vi "Client UI.vi"() -> ()   [LabVIEW 2020, in "LV Chat Client.lvclass"]
uses:
  LV Chat Client.lvclass
  UI State.ctl
  Data Types/Message.ctl
  LV Chat Client.lvclass/LV Chat Client.ctl
  <vilib>/IlluminatedG/lv-msg-simple/Stream-Simple-Msg/Manager/Manager.lvclass
  Data Types/Message ID.ctl
  <vilib>/event_ctls.llb/eventvkey.ctl
  Events.ctl
  <vilib>/IlluminatedG/lv-stream/Connection State.ctl
  Data Types/User Info.ctl
  01a2a97e-4748-4b48-9309-911c4d3a1048.vi
  b7fc8858-76c6-4de5-805f-2f843daa277e.vi
  b7fc8858-76c6-4de5-805f-2f843daa277e.vi/43e93f4b-eb60-4448-b7e4-56a49cc750fb.vi
  b7fc8858-76c6-4de5-805f-2f843daa277e.vi/0bdc4188-3073-475f-bdb7-d424a9377977.vi
  <vilib>/IlluminatedG/lv-msg-simple/Stream-Simple-Msg/Message/_Create.vi
  <vilib>/IlluminatedG/lv-msg-simple/Stream-Simple-Msg/Manager/Get Endpoints.vi
  <vilib>/IlluminatedG/lv-msg-simple/Stream-Simple-Msg/Message/Get Flattened Message.vi
  <vilib>/IlluminatedG/lv-msg-simple/Stream-Simple-Msg/Endpoint/Get Stream.vi
  <vilib>/IlluminatedG/lv-msg-simple/Stream-Simple-Msg/Message/Message.lvclass
  <vilib>/IlluminatedG/lv-stream/stream/Stream.lvclass
  <vilib>/IlluminatedG/lv-stream/Stream.lvlib
panel:
  in  "Timestamps":bool
  out "# Users":i32
  in  "Disconnect":bool
  in  "Connect":bool
  out "Log":string
  out "Users":i32(listbox)
  in  "Send":bool
  in  "Text":string
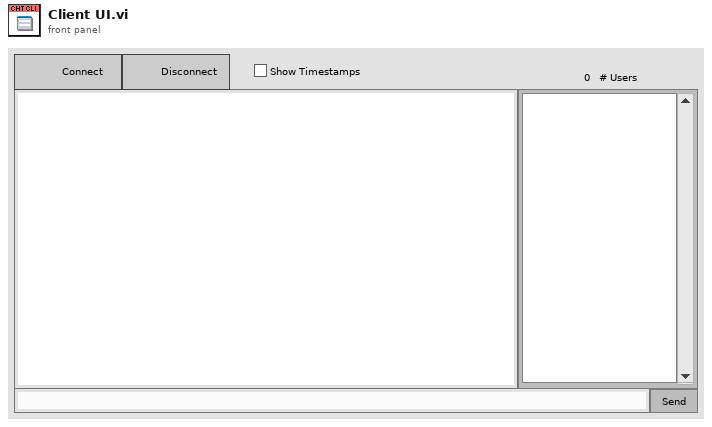
[diagram p1: front panel]
types:
  T1 = typedef "LV Chat Client.lvclass/UI State.ctl" = enum16{"Init", "Run", "Close"}
  T2 = typedef "Message.ctl" = cluster{"From":string, "Time":dbl, "Message":string}
  T3 = enum8{"Enabled", "Disabled", "Disabled and Grayed Out"}
  T4 = typedef "Message ID.ctl" = enum16{"UserInfo", "UserList", "Message", "Disconnect"}
  T5 = typedef "eventvkey.ctl" = enum16{"ASCII", "Enter", "Return", "Shift", "Ctrl", "Alt", "Cmd", "Opt", "Caps", "NumLock", "Clear", "Break", "Up", "Down", "Left", "Right", "Insert", "Delete", "Home", "End", "PageUp", "PageDown", "Escape", "Help", "Pause", "ScrollLock", "F1", "F2", "F3", "F4", "F5", "F6", "F7", "F8", "F9", "F10", "F11", "F12", "F13", "F14", "F15", "F16", "F17", "F18", "F19", "F20", "F21", "F22", "F23", "F24", "Play", "VolumeUp", "VolumeDown", "Mute", "Two Byte Char"}
  T6 = typedef "LV Chat Client.lvclass/Events.ctl" = cluster{"Userlist":refnum<user-event>, "Message":refnum<user-event>, "Prompt Name":refnum<user-event>, "Connection":refnum<user-event>, "Userinfo":refnum<user-event>, "Log":refnum<user-event>, "Update Log":refnum<user-event>}
  T7 = typedef "Stream.lvlib/Connection State.ctl" = enum16{"Connected", "Disconnected"}
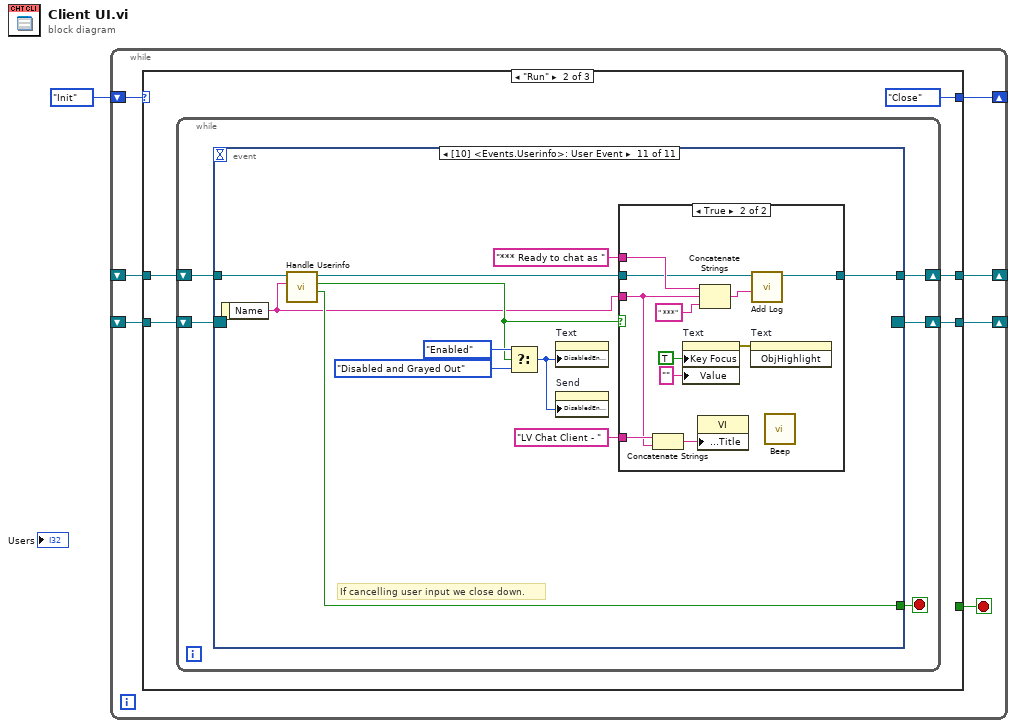
[diagram p0: block diagram]
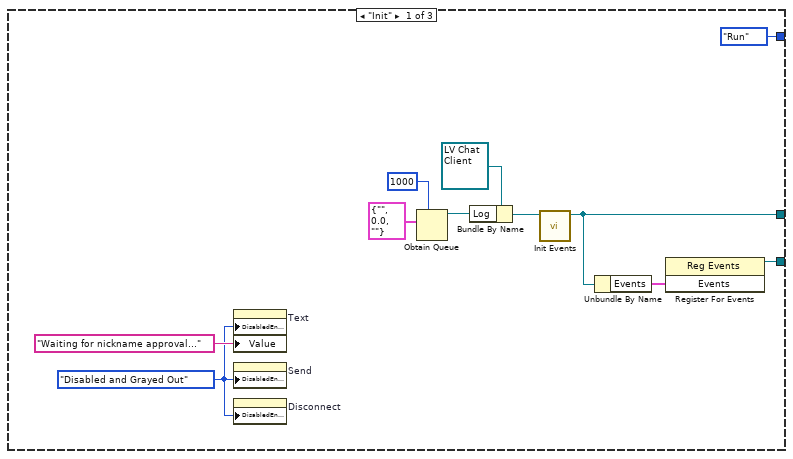
[diagram p2: hidden frame]
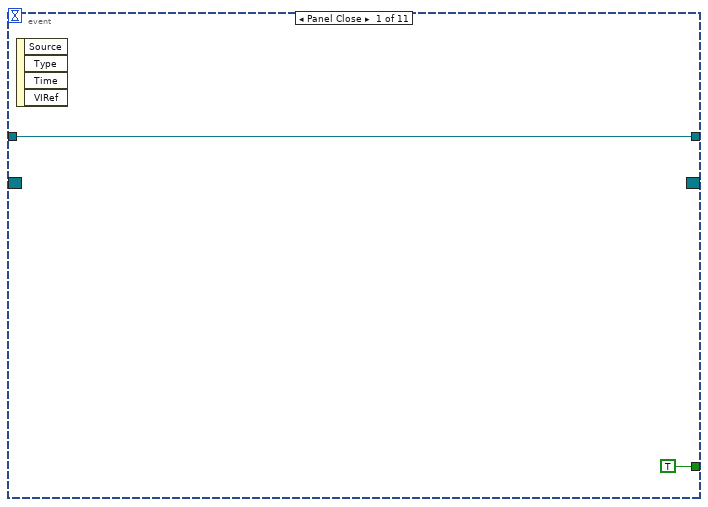
[diagram p3: hidden frame]
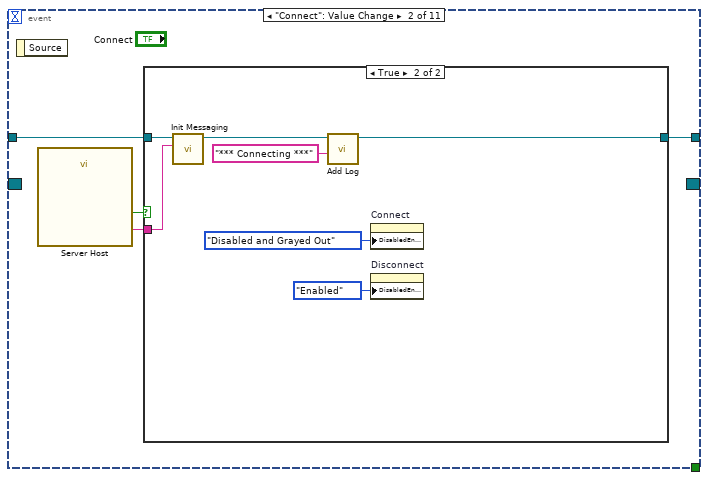
[diagram p4: hidden frame]
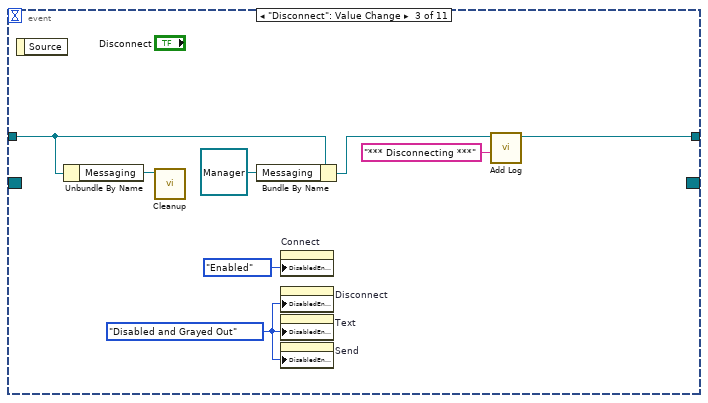
[diagram p6: hidden frame]
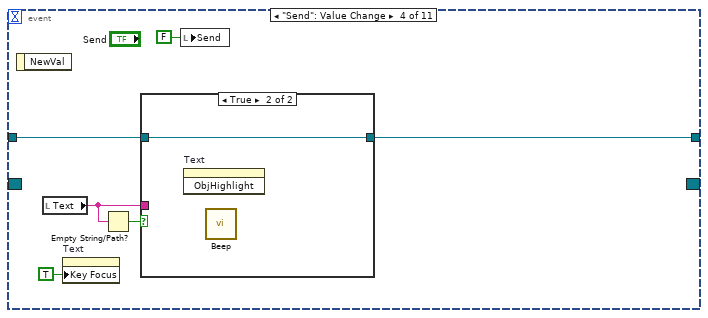
[diagram p7: hidden frame]
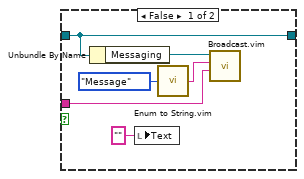
[diagram p8: hidden frame]
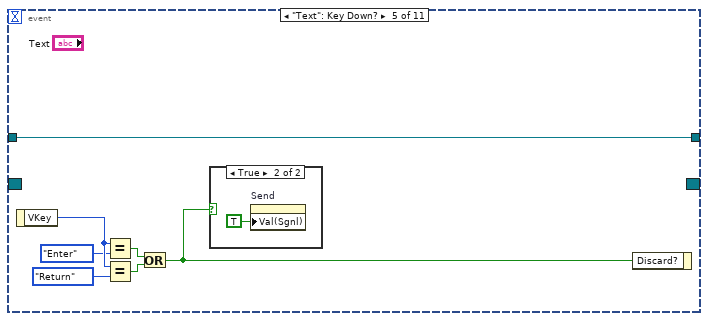
[diagram p9: hidden frame]
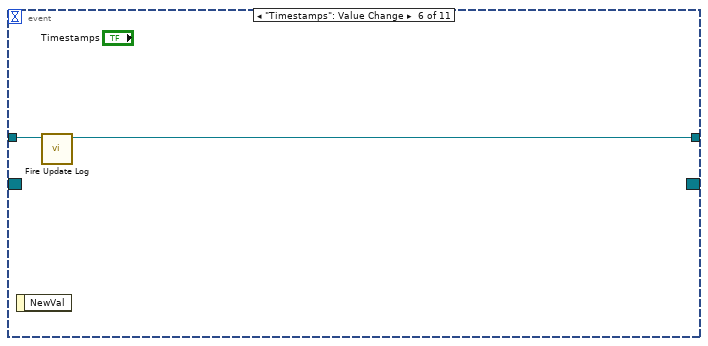
[diagram p11: hidden frame]
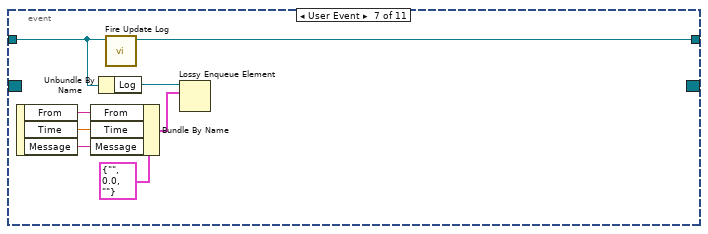
[diagram p12: hidden frame]
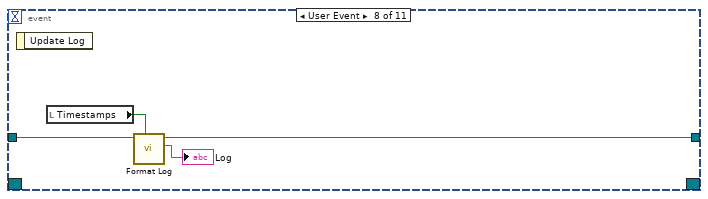
[diagram p13: hidden frame]
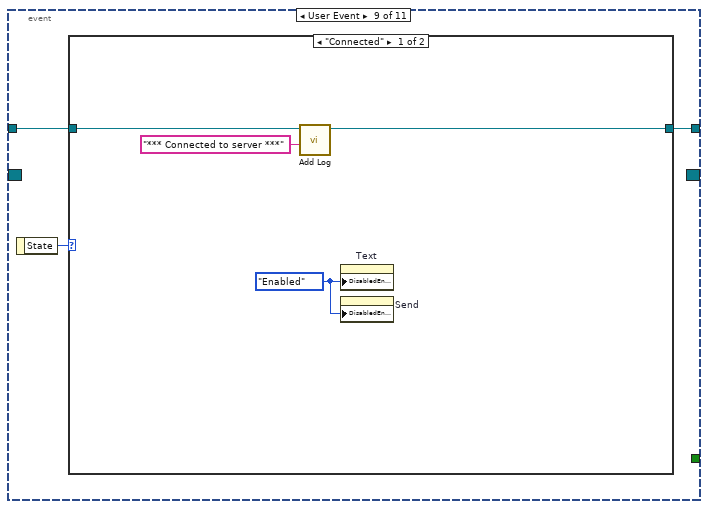
[diagram p14: hidden frame]
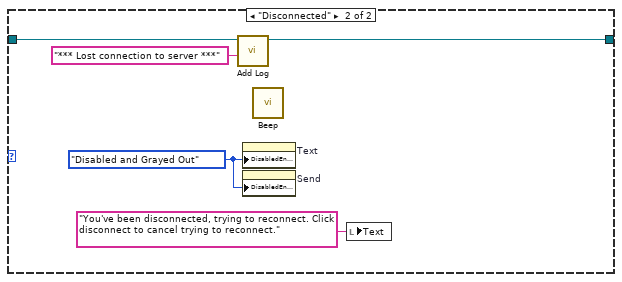
[diagram p15: hidden frame]
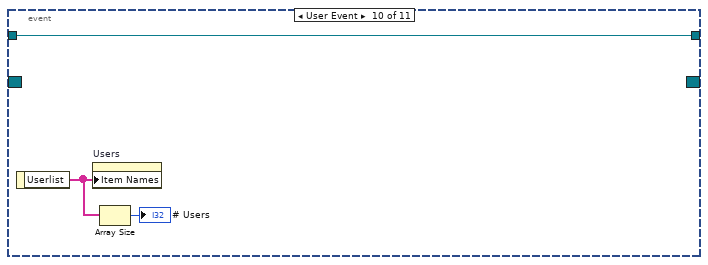
[diagram p16: hidden frame]
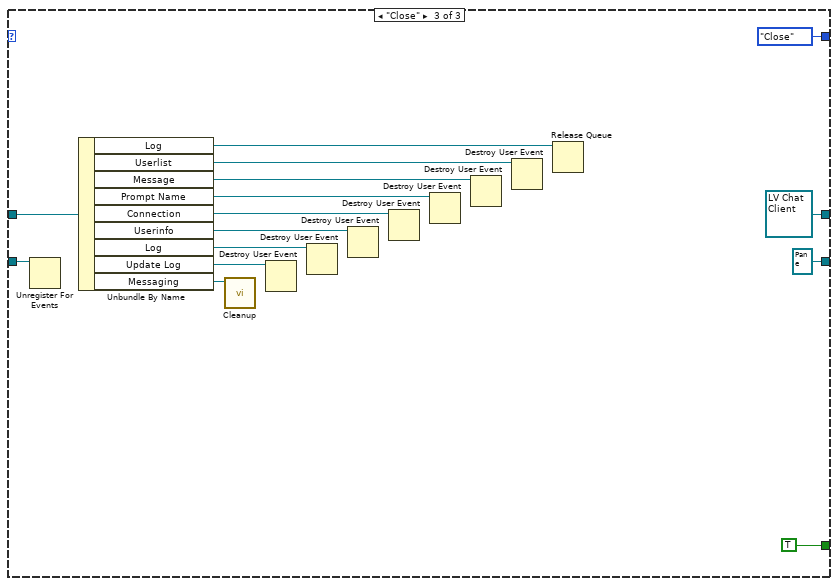
[diagram p18: hidden frame]
diagram:
  n1 = while {
    shift-right: [w5] -> _
    shift-left: UI_State."Init" ("UI State") -> [w8]
    shift-right: [w4] -> _
    shift-left: _ -> [w7]
    shift-right: [w3] -> _
    shift-left: _ -> [w2]
    stop <- w6 stop-if-true
    n2 = case shown="\"Run\"" w8 {
      tunnel: w7 -> [_ w23 w134]
      tunnel: [_ _ TRUE] -> w6
      tunnel: [UI_State."Run" ("UI State") UI_State."Close" ("UI State") UI_State."Close" ("UI State")] -> w5
      tunnel: [w13 w22 refnum<class "LV Chat Client.lvclass"> refnum ("LV Chat Client out")] -> w4
      tunnel: [w17 w20 refnum<event-registration> refnum ("Event Registration Refnum")] -> w3
      tunnel: w2 -> [_ w21 w136]
      frame "Init" {
        w15 = T3."Disabled and Grayed Out" ("Disabled")
        n3 = property on="Text" class="Str"("DisabledEnum"=w15, "Value"="Waiting for nickname approval..." ("Text")) -> ()  [unwired: 2 in, 2 out]
        n4 = property on="Send" class="Bool (strict)"("DisabledEnum"=w15) -> ()  [unwired: 2 in, 2 out]
        n5 = property on="Disconnect" class="Bool"("DisabledEnum"=w15) -> ()  [unwired: 2 in, 2 out]
        n6 = Obtain Queue(max queue size (-1, unlimited)=1000, element data type=T2 {"From"="", "Time"=0.0, "Message"=""} ("Message")) -> (queue out=w9:refnum<queue>)  [unwired: 3 in, 2 out]
        n7 = Bundle By Name(cluster=refnum<class "LV Chat Client.lvclass"> refnum ("LV Chat Client out"), "Log"=w9) -> (w12:refnum<class "LV Chat Client.lvclass">)
        n8 = call "Init Events.vi"("LV Chat Client in"=w12) -> ("LV Chat Client out"=w13:refnum<class "LV Chat Client.lvclass">)  [unwired: 9 in, 1 out]
        n9 = Unbundle By Name(w13) -> ("Events"=w18:T6)
        n10 = register-events(w18) -> (reference out=w17:refnum<event-registration>)  [unwired: 2 in, 1 out]
      }
      frame "Run" {
        n11 = while {
          shift-right: [w27] -> w22
          shift-left: w23 -> [w28]
          shift-right: [w25] -> w20
          shift-left: w21 -> [w26]
          stop <- w29 stop-if-true
          n12 = event shown="[10] <Events.Userinfo>: User Event" {
            selector: w26 -> [_ _ _ _ _ _ _ _ _ _ _]
            dyn-events: [_ _ _ _ _ _ _ _ _ _ _] -> w25
            timeout: _ -> [_ _ _ _ _ _ _ _ _ _ _]
            tunnel: [TRUE _ _ _ _ _ _ _ _ _ w111] -> w29
            tunnel: w28 -> [w30 w34 w49 w54 w65 w74 w76 w86 w88 w99 w112]
            tunnel: [w30 w32 w45 w53 w65 w73 w75 w84 w87 w99 w104] -> w27
            event Panel Close {
              n13 = event-data() -> ()  [unwired: 1 in, 4 out]
            }
            event "Connect": Value Change {
              n14 = event-data() -> ()  [unwired: 1 in, 1 out]
              n15 = call "Server Host"() -> ("Server Host"=w33:string, "OK"=w35:bool)  [unwired: 17 in, 1 out]
              n16 = case shown="True" w35 {
                tunnel: w34 -> [w36 w43]
                tunnel: w33 -> [_ w42]
                tunnel: [w36 w37] -> w32
                frame False {
                }
                frame True {
                  n17 = call "Init Messaging.vi"("Server Host"=w42, "LV Chat Client in"=w43) -> ("LV Chat Client out"=w39:refnum<class "LV Chat Client.lvclass">)  [unwired: 8 in, 1 out]
                  n18 = call "Add Log.vi"("Message"="*** Connecting ***", "LV Chat Client in"=w39) -> ("LV Chat Client out"=w37:refnum<class "LV Chat Client.lvclass">)  [unwired: 8 in, 1 out]
                  n19 = property on="Connect" class="Bool"("DisabledEnum"=T3."Disabled and Grayed Out" ("Disabled")) -> ()  [unwired: 2 in, 2 out]
                  n20 = property on="Disconnect" class="Bool"("DisabledEnum"=T3."Enabled" ("Disabled")) -> ()  [unwired: 2 in, 2 out]
                }
              }
            }
            event "Disconnect": Value Change {
              w47 = T3."Disabled and Grayed Out" ("Disabled")
              n21 = event-data() -> ()  [unwired: 1 in, 1 out]
              n22 = Unbundle By Name(w49) -> ("Messaging"=w50:refnum<class "Manager.lvclass">)
              n23 = call <vilib>:"Cleanup.vi"("Manager in"=w50) -> ()  [unwired: 10 in, 1 out]
              n24 = Bundle By Name(cluster=w49, "Messaging"=refnum<class "Manager.lvclass"> refnum) -> (w46:refnum<class "LV Chat Client.lvclass">)
              n25 = property on="Connect" class="Bool"("DisabledEnum"=T3."Enabled" ("Disabled")) -> ()  [unwired: 2 in, 2 out]
              n26 = property on="Disconnect" class="Bool"("DisabledEnum"=w47) -> ()  [unwired: 2 in, 2 out]
              n27 = property on="Text" class="Str"("DisabledEnum"=w47) -> ()  [unwired: 2 in, 2 out]
              n28 = property on="Send" class="Bool (strict)"("DisabledEnum"=w47) -> ()  [unwired: 2 in, 2 out]
              n29 = call "Add Log.vi"("Message"="*** Disconnecting ***", "LV Chat Client in"=w46) -> ("LV Chat Client out"=w45:refnum<class "LV Chat Client.lvclass">)  [unwired: 8 in, 1 out]
            }
            event "Send": Value Change {
              n30 = event-data() -> ()  [unwired: 1 in, 1 out]
              n31 = local read "Text"() -> (w55:string)
              n32 = property on="Text" class="Str"("Key Focus"=TRUE) -> ()  [unwired: 2 in, 2 out]
              n33 = Empty String/Path?(string/path=w55) -> (empty?=w56:bool)
              n34 = case shown="True" w56 {
                tunnel: w55 -> [w60 _]
                tunnel: w54 -> [w62 w64]
                tunnel: [w62 w64] -> w53
                frame False {
                  n35 = Unbundle By Name(w62) -> ("Messaging"=w61:refnum<class "Manager.lvclass">)
                  n36 = local write "Text"("" ("Text")) -> ()
                  n37 = call "Enum to String.vim"("Enum"=Message_ID."Message" ("Message ID")) -> ("Enum String"=w58:string)
                  n38 = call "Broadcast.vim"("Data (With ID String)"=w60, "Message (Or ID String)"=w58, "Manager in"=w61) -> ()  [unwired: 7 in, 2 out]
                }
                frame True {
                  n39 = invoke on="Text" class="Str" method="ObjHighlight"() -> ()  [unwired: 3 in, 3 out]
                  n40 = call <vilib>:"Beep.vi"() -> ()  [unwired: 12 in]
                }
              }
              n41 = local write "Send"(FALSE ("Send")) -> ()
            }
            event "Text": Key Down? {
              n42 = event-data() -> ("VKey"=w71:T5)  [unwired: 1 in]
              n43 = Equal?(x=w71, y=eventvkey."Enter") -> (x = y?=w68:bool)
              n44 = Equal?(x=w71, y=eventvkey."Return") -> (x = y?=w67:bool)
              n45 = Or(x=w68, y=w67) -> (x .or. y?=w66:bool)
              n46 = case shown="True" w66 {
                frame False {
                }
                frame True {
                  n47 = property on="Send" class="Bool (strict)"("Val(Sgnl)"=TRUE ("Value (Signaling)")) -> ()  [unwired: 2 in, 2 out]
                }
              }
              n48 = event-data("Discard?"=w66) -> ()  [unwired: 1 in, 1 out]
            }
            event "Timestamps": Value Change {
              n49 = event-data() -> ()  [unwired: 1 in, 1 out]
              n50 = call "Fire Update Log.vi"("LV Chat Client in"=w74) -> ("LV Chat Client out"=w73:refnum<class "LV Chat Client.lvclass">)  [unwired: 9 in, 1 out]
            }
            event User Event {
              n51 = event-data() -> ("From"=w81:string, "Time"=w80:dbl, "Message"=w79:string)  [unwired: 1 in]
              n52 = Bundle By Name(cluster=T2 {"From"="", "Time"=0.0, "Message"=""} ("Message"), "From"=w81, "Time"=w80, "Message"=w79) -> (w77:T2)
              n53 = Unbundle By Name(w76) -> ("Log"=w78:refnum<queue>)
              n54 = call "Fire Update Log.vi"("LV Chat Client in"=w76) -> ("LV Chat Client out"=w75:refnum<class "LV Chat Client.lvclass">)  [unwired: 9 in, 1 out]
              n55 = Lossy Enqueue Element(queue=w78, element=w77) -> ()  [unwired: 1 in, 4 out]
            }
            event User Event {
              n56 = event-data() -> ()  [unwired: 1 in, 1 out]
              n57 = local read "Timestamps"() -> (w85:bool)
              n58 = call "Format Log.vi"("Show Timestamps"=w85, "LV Chat Client in"=w86) -> ("Log"=→"Log":string, "LV Chat Client out"=w84:refnum<class "LV Chat Client.lvclass">)  [unwired: 7 in, 1 out]
            }
            event User Event {
              n59 = event-data() -> ("State"=w89:T7)  [unwired: 1 in]
              n60 = case shown="\"Connected\"" w89 {
                tunnel: w88 -> [w92 w96]
                tunnel: [w90 w94] -> w87
                frame "Connected" {
                  w93 = T3."Enabled" ("Disabled")
                  n61 = call "Add Log.vi"("Message"="*** Connected to server ***", "LV Chat Client in"=w92) -> ("LV Chat Client out"=w90:refnum<class "LV Chat Client.lvclass">)  [unwired: 8 in, 1 out]
                  n62 = property on="Text" class="Str"("DisabledEnum"=w93) -> ()  [unwired: 2 in, 2 out]
                  n63 = property on="Send" class="Bool (strict)"("DisabledEnum"=w93) -> ()  [unwired: 2 in, 2 out]
                }
                frame "Disconnected" {
                  w98 = T3."Disabled and Grayed Out" ("Disabled")
                  n64 = call "Add Log.vi"("Message"="*** Lost connection to server ***", "LV Chat Client in"=w96) -> ("LV Chat Client out"=w94:refnum<class "LV Chat Client.lvclass">)  [unwired: 8 in, 1 out]
                  n65 = property on="Text" class="Str"("DisabledEnum"=w98) -> ()  [unwired: 2 in, 2 out]
                  n66 = property on="Send" class="Bool (strict)"("DisabledEnum"=w98) -> ()  [unwired: 2 in, 2 out]
                  n67 = call <vilib>:"Beep.vi"() -> ()  [unwired: 12 in]
                  n68 = local write "Text"("You've been disconnected, trying to reconnect. Click disconnect to cancel trying to reconnect." ("Text")) -> ()
                }
              }
            }
            event User Event {
              n69 = event-data() -> ("Userlist"=w101:string[])  [unwired: 1 in]
              n70 = property on="Users" class="LstBox (strict)"("Item Names"=w101) -> ()  [unwired: 2 in, 2 out]
              n71 = Array Size(array=w101) -> (size(s)=→"# Users":i32)
            }
            event User Event {
              # "If cancelling user input we close down."
              n72 = event-data() -> ("Name"=w106:string)  [unwired: 1 in]
              n73 = call "Handle Userinfo.vi"("Name"=w106, "LV Chat Client in"=w112) -> ("Cancelled?"=w111:bool, "Name Accepted?"=w108:bool, "LV Chat Client out"=w107:refnum<class "LV Chat Client.lvclass">)  [unwired: 6 in, 1 out]
              n74 = Select(t=T3."Enabled" ("Disabled"), s=w108, f=T3."Disabled and Grayed Out" ("Disabled")) -> (s? t:f=w103:T3)
              n75 = property on="Text" class="Str"("DisabledEnum"=w103) -> ()  [unwired: 2 in, 2 out]
              n76 = property on="Send" class="Bool (strict)"("DisabledEnum"=w103) -> ()  [unwired: 2 in, 2 out]
              n77 = case shown="True" w108 {
                tunnel: w107 -> [w113 w119]
                tunnel: w106 -> [_ w115]
                tunnel: "*** Ready to chat as " -> [_ w121]
                tunnel: [w113 w117] -> w104
                tunnel: "LV Chat Client - " -> [_ w116]
                frame False {
                }
                frame True {
                  n78 = Concatenate Strings(w116, w115) -> (w114:string)
                  n79 = property on="Text" class="Str"("Key Focus"=TRUE, "Value"="" ("Text")) -> (error out=w123:errorcluster)  [unwired: 2 in, 1 out]
                  n80 = property class="VI"("Front Panel.Title"=w114) -> ()  [unwired: 2 in, 2 out]
                  n81 = Concatenate Strings(w121, w115, " ***" ("string")) -> (w118:string)
                  n82 = invoke on="Text" class="Str" method="ObjHighlight"(error in=w123) -> ()  [unwired: 2 in, 3 out]
                  n83 = call "Add Log.vi"("Message"=w118, "LV Chat Client in"=w119) -> ("LV Chat Client out"=w117:refnum<class "LV Chat Client.lvclass">)  [unwired: 8 in, 1 out]
                  n84 = call <vilib>:"Beep.vi"() -> ()  [unwired: 12 in]
                }
              }
            }
          }
        }
      }
      frame "Close" {
        n85 = Unregister For Events(event registration refnum=w136) -> ()  [unwired: 1 in, 1 out]
        n86 = Unbundle By Name(w134) -> ("Log"=w125:refnum<queue>, "Userlist"=w126:refnum<user-event>, "Message"=w127:refnum<user-event>, "Prompt Name"=w128:refnum<user-event>, "Connection"=w129:refnum<user-event>, "Userinfo"=w130:refnum<user-event>, "Log"=w131:refnum<user-event>, "Update Log"=w132:refnum<user-event>, "Messaging"=w133:refnum<class "Manager.lvclass">)
        n87 = call <vilib>:"Cleanup.vi"("Manager in"=w133) -> ()  [unwired: 10 in, 1 out]
        n88 = Destroy User Event(user event=w132) -> ()  [unwired: 1 in, 1 out]
        n89 = Destroy User Event(user event=w131) -> ()  [unwired: 1 in, 1 out]
        n90 = Destroy User Event(user event=w130) -> ()  [unwired: 1 in, 1 out]
        n91 = Destroy User Event(user event=w129) -> ()  [unwired: 1 in, 1 out]
        n92 = Destroy User Event(user event=w128) -> ()  [unwired: 1 in, 1 out]
        n93 = Destroy User Event(user event=w127) -> ()  [unwired: 1 in, 1 out]
        n94 = Destroy User Event(user event=w126) -> ()  [unwired: 1 in, 1 out]
        n95 = Release Queue(queue=w125) -> ()  [unwired: 2 in, 3 out]
      }
    }
  }
